vi "Get Adjacents.vi"(9 "Column":i32, 10 "Row":i32, 11 "Array":u8[][](array[numeric])) -> (1 "Columns Out":i32[](array[numeric]), 2 "Rows Out":i32[](array[numeric]), 3 "Values":u8[](array[numeric]))   [LabVIEW 2019, in "Day 15.lvlib"]
uses:
  Day 15.lvlib
  Controls/Side.ctl
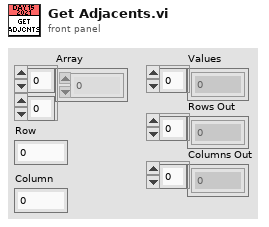
[diagram p1: front panel]
types:
  T1 = typedef "Day 15.lvlib/Side.ctl" = enum16{"Rigth", "Left", "Down", "Up", "Rigth Up", "Rigth Down", "Left Up", "Left Down"}
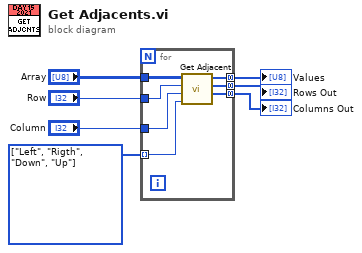
[diagram p0: block diagram]
diagram:
  w4 = T1[] [enum."Left", enum."Rigth", enum."Down", enum."Up"] items=["Rigth", "Left", "Down", "Up", "Rigth Up", "Rigth Down", "Left Up", "Left Down"]
  n1 = for {
    tunnel: "Array" -> [w14]
    tunnel: w4 -> [w11] mode=indexing
    tunnel: "Row" -> [w13]
    tunnel: "Column" -> [w12]
    tunnel: [w10] -> w3 mode=concatenating
    tunnel: [w9] -> w2 mode=concatenating
    tunnel: [w8] -> w1 mode=concatenating
    n2 = call "Get Adjacent.vi"("Side"=w11, "Column In"=w12, "Row In"=w13, "Array In"=w14) -> ("Column Out"=w8:i32[], "Row Out"=w9:i32[], "Array"=w10:u8[])  [unwired: 5 in]
  }
  "Values" <- w3
  "Rows Out" <- w2
  "Columns Out" <- w1
